vi "Execute Initial Value Policy.vi"(8 "error in (no error)":errorcluster, 9 "Last Publish Time":timestamp, 10 "Last Topic Value":variant, 11 "WriteWhenVisibleSubscription In":refnum<class "WriteWhenVisibleSubscription.lvclass">) -> (0 "error out":errorcluster, 3 "WriteWhenVisibleSubscription Out":refnum<class "WriteWhenVisibleSubscription.lvclass">)   [LabVIEW 2019, in "SubscriptionPolicy.lvlib" / "WriteWhenVisibleSubscription.lvclass"]
uses:
  <vilib>/gpm_packages/@cs/mva-core/Source/SubscriptionPolicy/WriteWhenVisibleSubscription/WriteWhenVisibleSubscription.lvclass
  <vilib>/gpm_packages/@cs/mva-core/Source/SubscriptionPolicy/WriteWhenVisibleSubscription/WriteWhenVisibleSubscription.lvclass/WriteWhenVisibleSubscription.ctl
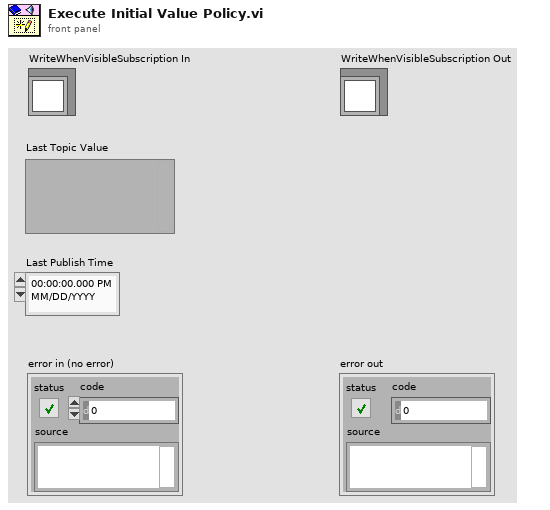
[diagram p1: front panel]
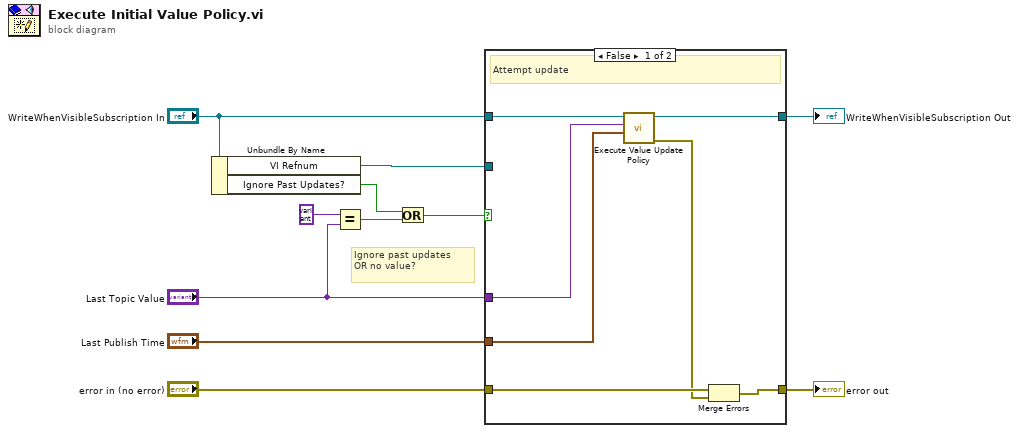
[diagram p0: block diagram]
diagram:
  # "Ignore past updates\nOR no value?"
  n1 = Unbundle By Name("WriteWhenVisibleSubscription In") -> ("VI Refnum"=w1:refnum<vi>, "Ignore Past Updates?"=w4:bool)
  n2 = Equal?(x=variant, y="Last Topic Value") -> (x = y?=w5:bool)
  n3 = Or(x=w4, y=w5) -> (x .or. y?=w3:bool)
  n4 = case shown="False" w3 {
    tunnel: "error in (no error)" -> [w18 w19]
    tunnel: "Last Topic Value" -> [w13 _]
    tunnel: "Last Publish Time" -> [w12 _]
    tunnel: [w17 w19] -> w9
    tunnel: "WriteWhenVisibleSubscription In" -> [w16 w20]
    tunnel: [w15 w20] -> w8
    tunnel: w1 -> [_ _]
    frame False {
      # "Attempt update"
      n5 = call-dynamic "Execute Value Update Policy.vi"("Publish Time"=w12, "New Topic Value"=w13, "WriteWhenVisibleSubscription In"=w16) -> ("error out"=w14:errorcluster, "WriteWhenVisibleSubscription Out"=w15:refnum<class "WriteWhenVisibleSubscription.lvclass">)  [unwired: 7 in]
      n6 = Merge Errors(w18, w14) -> (w17:errorcluster)
    }
    frame True {
      # "Do not update"
    }
  }
  "error out" <- w9
  "WriteWhenVisibleSubscription Out" <- w8
